vi "NumatoRelay.FG Simple RelayBrd Controller.vi"(6 "PID":string="0C06", 7 "VisaTimeout":u32=2000, 8 "VID":string="2A19", 9 "State":bool, 10 "IO Num":i32 min=0 max=3 step=1, 11 "Action":T1(ring)) -> (0 "error out":errorcluster, 3 "State Out":bool)   [LabVIEW 2018]
uses:
  <vilib>/Instr/_visa.llb/VISA Configure Serial Port (Instr).vi
  <vilib>/KATE/Time/Time Utils.lvlib
panel:
  out "Cmd":string
  out "ReadData":string
  out "VISA Name":refnum<visa-resource-name>
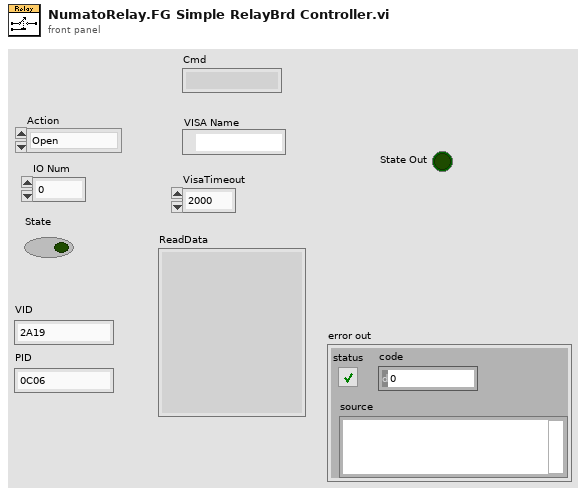
[diagram p1: front panel]
types:
  T1 = enum16{"Open", "Set Relay", "Read GPIO", "Close"}
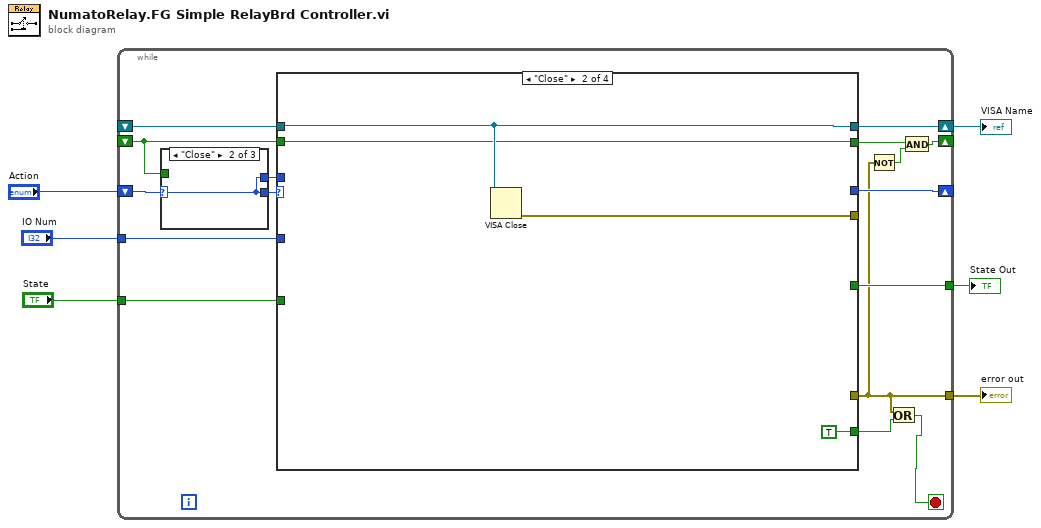
[diagram p0: block diagram]
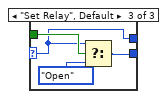
[diagram p3: hidden frame]
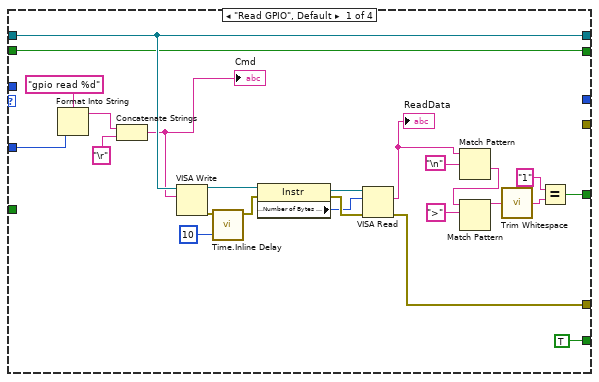
[diagram p4: hidden frame]
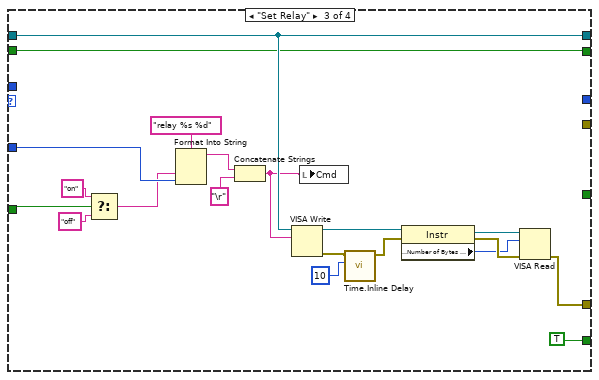
[diagram p5: hidden frame]
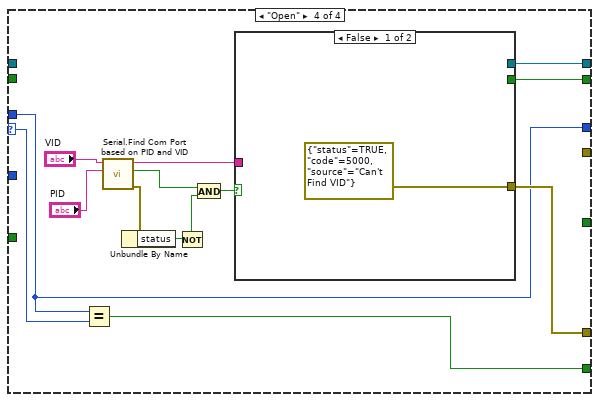
[diagram p6: hidden frame]
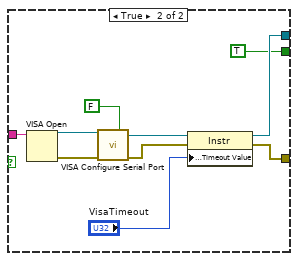
[diagram p7: hidden frame]
diagram:
  n1 = while {
    shift-right: [w21] -> w2
    shift-left: _ -> [w22]
    tunnel: [w13] -> w6
    tunnel: "IO Num" -> [w20]
    tunnel: "State" -> [w19]
    tunnel: [w18] -> w3
    shift-right: [w17] -> _
    shift-left: _ -> [w7]
    shift-right: [w14] -> _
    shift-left: "Action" -> [w10]
    stop <- w11 stop-if-true
    n2 = case shown="\"Close\"" w10 {
      selector: w10 -> [w23 w24 w25]
      tunnel: [w23 w24 w28] -> w9
      tunnel: [w23 w24 w25] -> w8
      tunnel: w7 -> [_ _ w27]
      frame "Open" {
      }
      frame "Close" {
      }
      frame "Set Relay", Default {
        n3 = Select(t=w25, s=w27, f=T1."Open") -> (s? t:f=w28:T1)
      }
    }
    n4 = case shown="\"Close\"" w9 {
      selector: w9 -> [_ _ _ w79]
      tunnel: w22 -> [w50 w56 w73 _]
      tunnel: [w50 w56 w73 w82] -> w21
      tunnel: [_ w55 _ _] -> _
      tunnel: [w34 _ w67 w81] -> w13
      tunnel: w20 -> [w47 _ w72 _]
      tunnel: w19 -> [_ _ w69 _]
      tunnel: [w40 _ _ _] -> w18
      tunnel: w7 -> [w30 w54 w58 _]
      tunnel: [w30 w54 w58 w80] -> w16
      tunnel: w8 -> [_ _ _ w77]
      tunnel: [TRUE TRUE TRUE w78] -> w12
      tunnel: [_ _ _ w77] -> w14
      frame "Read GPIO", Default {
        n5 = Format Into String(format string="gpio read %d", w47) -> (resulting string=w52:string)  [unwired: 2 in, 1 out]
        n6 = Concatenate Strings(w52, "\r") -> (w49:string)
        "Cmd" <- w49
        n7 = VISA Write(VISA resource name=w50, write buffer=w49) -> (VISA resource name out=w36:refnum<visa-resource-name>, error out=w32:errorcluster)  [unwired: 1 in, 1 out]
        n8 = call <vilib>:"Time.Inline Delay.vi"("Wait(ms)"=u32 10, "error in top"=w32) -> ("error out top"=w33:errorcluster)  [unwired: 8 in, 1 out]
        n9 = property class="Instr"(reference=w36, error in=w33) -> (reference out=w38:refnum<visa-resource-name>, error out=w39:errorcluster, "Serial Settings:Number of Bytes at Serial Port"=w37:u32)
        n10 = VISA Read(VISA resource name=w38, byte count=w37, error in (no error)=w39) -> (read buffer=w35:string, error out=w34:errorcluster)  [unwired: 2 out]
        "ReadData" <- w35
        n11 = Match Pattern(string=w35, regular expression="\n") -> (after substring=w45:string)  [unwired: 1 in, 3 out]
        n12 = Match Pattern(string=w45, regular expression=">") -> (before substring=w43:string)  [unwired: 1 in, 3 out]
        n13 = call <vilib>:"Trim Whitespace.vi"("string"=w43) -> ("trimmed string"=w42:string)  [unwired: 1 in]
        n14 = Equal?(x="1", y=w42) -> (x = y?=w40:bool)
      }
      frame "Close" {
        n15 = VISA Close(VISA resource name=w56) -> (error out=w55:errorcluster)  [unwired: 1 in]
      }
      frame "Set Relay" {
        n16 = Select(t="on", s=w69, f="off") -> (s? t:f=w68:string)
        n17 = Format Into String(format string="relay %s %d", w68, w72) -> (resulting string=w76:string)  [unwired: 2 in, 1 out]
        n18 = Concatenate Strings(w76, "\r") -> (w66:string)
        n19 = VISA Write(VISA resource name=w73, write buffer=w66) -> (VISA resource name out=w65:refnum<visa-resource-name>, error out=w61:errorcluster)  [unwired: 1 in, 1 out]
        n20 = local write "Cmd"(w66) -> ()
        n21 = call <vilib>:"Time.Inline Delay.vi"("Wait(ms)"=u32 10, "error in top"=w61) -> ("error out top"=w60:errorcluster)  [unwired: 8 in, 1 out]
        n22 = property class="Instr"(reference=w65, error in=w60) -> (reference out=w63:refnum<visa-resource-name>, error out=w64:errorcluster, "Serial Settings:Number of Bytes at Serial Port"=w62:u32)
        n23 = VISA Read(VISA resource name=w63, byte count=w62, error in (no error)=w64) -> (error out=w67:errorcluster)  [unwired: 3 out]
      }
      frame "Open" {
        n24 = Equal?(x=w77, y=w79) -> (x = y?=w78:bool)
        n25 = call "Serial.Find Com Port based on PID and VID.vi"("PID"="PID", "VID"="VID") -> ("error out"=w90:errorcluster, "Found"=w89:bool, "COM Port"=w85:string)  [unwired: 5 in, 2 out]
        n26 = Unbundle By Name(w90) -> ("status"=w88:bool)
        n27 = Not(x=w88) -> (.not. x?=w87:bool)
        n28 = And(x=w89, y=w87) -> (x .and. y?=w86:bool)
        n29 = case shown="False" w86 {
          tunnel: w85 -> [_ w101]
          tunnel: [_ w95] -> w82
          tunnel: [errorcluster {"status"=TRUE, "code"=5000, "source"="Can't Find VID"} ("error constant") w94] -> w81
          tunnel: [_ TRUE] -> w80
          frame False {
          }
          frame True {
            n30 = VISA Open(VISA resource name=w101) -> (VISA resource name=w100:refnum<visa-resource-name>, error out=w99:errorcluster)  [unwired: 4 in]
            n31 = call-poly "VISA Configure Serial Port"("VISA resource name"=w100, "Enable Termination\nChar (T)"=FALSE ("Enable Termination\nChar (T)"), "error in (no error)"=w99) -> ("VISA resource name out"=w96:refnum<visa-resource-name>, "error out"=w93:errorcluster)  [unwired: 11 in]
            n32 = property class="Instr"(reference=w96, error in=w93, "General Settings:Timeout Value"="VisaTimeout") -> (reference out=w95:refnum<visa-resource-name>, error out=w94:errorcluster)
          }
        }
      }
    }
    n33 = Not(x=w13) -> (.not. x?=w15:bool)
    n34 = Or(x=w13, y=w12) -> (x .or. y?=w11:bool)
    n35 = And(x=w16, y=w15) -> (x .and. y?=w17:bool)
  }
  "error out" <- w6
  "State Out" <- w3
  "VISA Name" <- w2
